vi "Get State from Mouse Coords over State String.vi"(8 "error in (no error)":errorcluster, 10 "Mouse Position":T1, 11 "StringConstant in":refnum<vi>) -> (0 "error out":errorcluster, 3 "State (entire line)":string)   [LabVIEW 2020]
uses:
  <vilib>/Utility/miscctls.llb/LVPositionTypeDef.ctl
  <userlib>/_OpenG.lib/string/string.llb/openg_string.lvlib
panel:
  out "Row":dbl
  out "Row (Rounded)":dbl
  out "Position":T1
  out "reference out":refnum<vi>
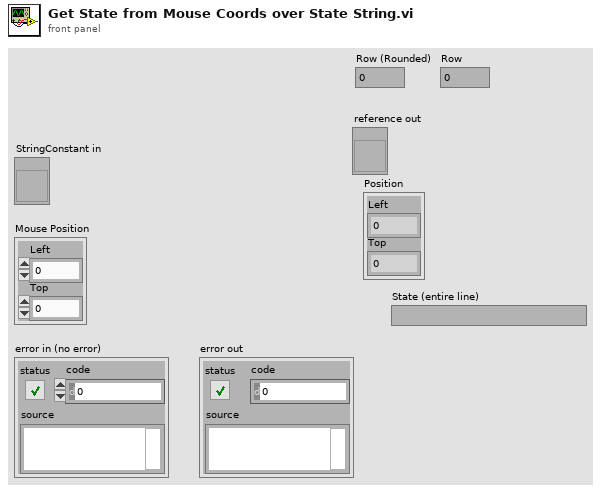
[diagram p1: front panel]
types:
  T1 = typedef "LVPositionTypeDef.ctl" = cluster{"Left":i32, "Top":i32}
  T2 = cluster{"Font Name:":string, "Size":i16, "Strikeout?":bool, "Italic?":bool, "Underline?":bool, "Outline?":bool, "Shadow?":bool, "Bold?":bool}
  T3 = enum16{"User-specified Font", "Application Font", "System Font", "Dialog Font"}
  T4 = typedef "LVFontTypeDef.ctl" = cluster{"Font Name":string, "Size":u16, "Bold":bool, "Italic":bool, "Underline":bool, "Strikeout":bool, "Color":u32}
  T5 = cluster{"left":i16, "top":i16, "right":i16, "bottom":i16}
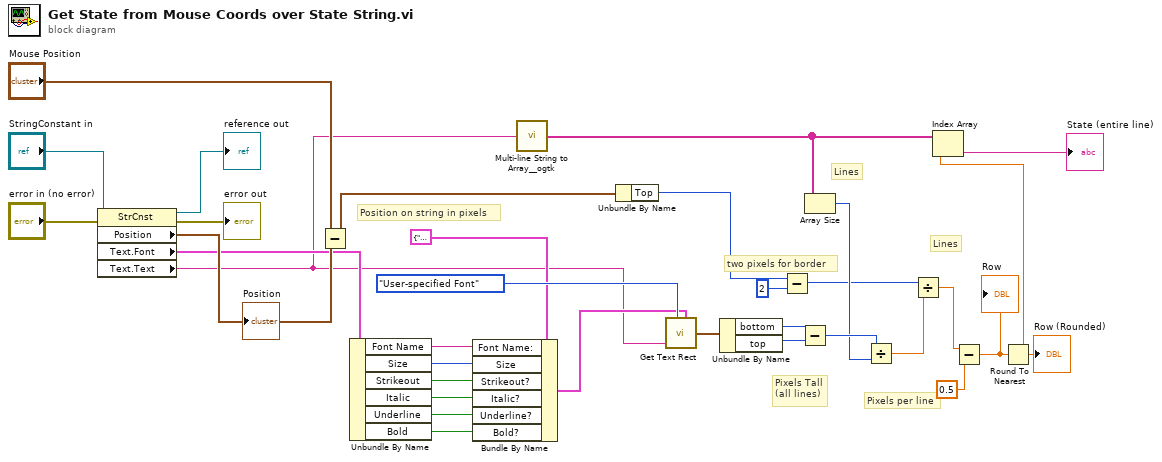
[diagram p0: block diagram]
diagram:
  # "two pixels for border"
  # "Lines"
  # "Pixels per line"
  # "Pixels Tall\n(all lines)"
  # "Lines"
  # "Position on string in pixels"
  n1 = property class="StrCnst"(reference="StringConstant in", error in="error in (no error)") -> (reference out=→"reference out":refnum<vi>, error out=→"error out":errorcluster, "Position"=w28:T1, "Text.Font"=w26:T4, "Text.Text"=w11:string)
  "Position" <- w28
  n2 = Subtract(x="Mouse Position", y=w28) -> (x-y=w17:T1)
  n3 = Unbundle By Name(w26) -> ("Font Name"=w24:string, "Size"=w23:u16, "Strikeout"=w22:bool, "Italic"=w21:bool, "Underline"=w20:bool, "Bold"=w19:bool)
  n4 = Bundle By Name(cluster=T2 {"Font Name:"="", "Size"=0, "Strikeout?"=FALSE, "Italic?"=FALSE, "Underline?"=FALSE, "Outline?"=FALSE, "Shadow?"=FALSE, "Bold?"=FALSE} ("[user-specified font]"), "Font Name:"=w24, "Size"=w23, "Strikeout?"=w22, "Italic?"=w21, "Underline?"=w20, "Bold?"=w19) -> (w18:T2)
  n5 = call <userlib>:"Multi-line String to Array__ogtk.vi"("string"=w11) -> ("lines"=w8:string[])
  n6 = Unbundle By Name(w17) -> ("Top"=w5:i32)
  n7 = call <vilib>:"Get Text Rect.vi"("desired font(Application)"=T3."User-specified Font", "text"=w11, "[user-specified font]"=w18) -> ("rect"=w16:T5)  [unwired: 6 in]
  n8 = Unbundle By Name(w16) -> ("bottom"=w15:i16, "top"=w14:i16)
  n9 = Subtract(x=w5, y=2 ("x")) -> (x-y=w2:i32)
  n10 = Subtract(x=w15, y=w14) -> (x-y=w7:i16)
  n11 = Array Size(array=w8) -> (size(s)=w6:i32)
  n12 = Divide(x=w7, y=w6) -> (x/y=w4:dbl)
  n13 = Divide(x=w2, y=w4) -> (x/y=w3:dbl)
  n14 = Subtract(x=w3, y=0.5) -> (x-y=w12:dbl)
  "Row" <- w12
  n15 = Round To Nearest(number=w12) -> (nearest integer value=w9:dbl)
  "Row (Rounded)" <- w9
  n16 = Index Array(array=w8, index=w9) -> (element=→"State (entire line)":string)
